vi "DecodeISAStatus.vi"(8 "error in (no error)":errorcluster, 11 "Message":string) -> (0 "error out":errorcluster, 1 "output cluster":T1, 2 "Pressure":dbl, 3 "IMP":i32, 5 "PWM":i32)   [LabVIEW 2017]
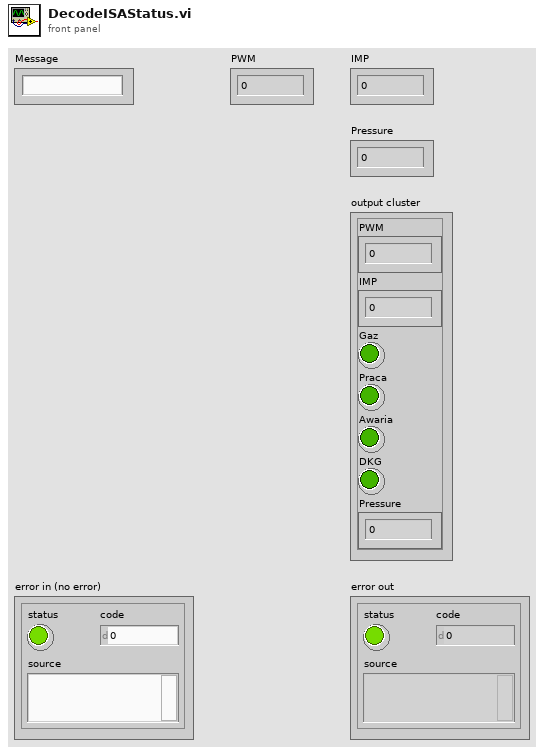
[diagram p1: front panel]
types:
  T1 = cluster{"PWM":i32, "IMP":i32, "Gaz":bool, "Praca":bool, "Awaria":bool, "DKG":bool, "Pressure":dbl}
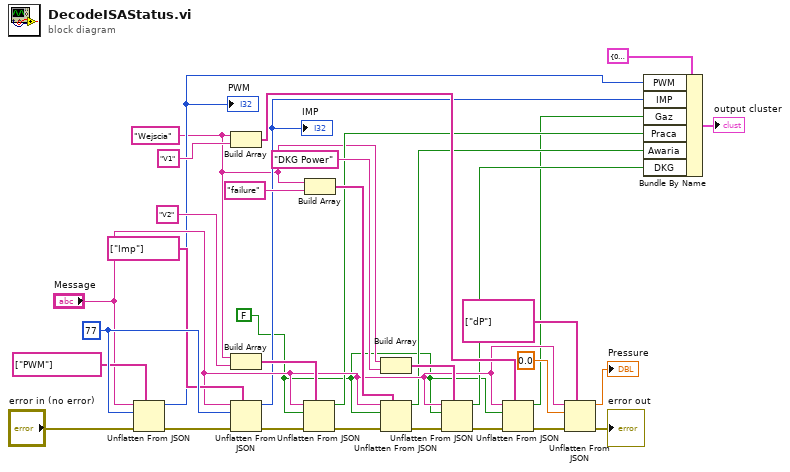
[diagram p0: block diagram]
diagram:
  w1 = FALSE
  w2 = "Wejscia"
  w30 = 77
  n1 = Unflatten From JSON(path=string[] ["PWM"], JSON string="Message", type and defaults=w30, error in (no error)="error in (no error)") -> (value=w11:i32, error out=w27:errorcluster)  [unwired: 3 in]
  "PWM" <- w11
  n2 = Build Array(w2, "V1" ("element")) -> (w14:string[])
  n3 = Build Array(w2, "V2" ("element")) -> (w17:string[])
  n4 = Unflatten From JSON(path=string[] ["Imp"], JSON string="Message", type and defaults=w30, error in (no error)=w27) -> (value=w10:i32, error out=w29:errorcluster)  [unwired: 3 in]
  "IMP" <- w10
  n5 = Unflatten From JSON(path=w17, JSON string="Message", type and defaults=w1, error in (no error)=w29) -> (value=w8:bool, error out=w25:errorcluster)  [unwired: 3 in]
  n6 = Build Array(w2, "failure" ("element")) -> (w16:string[])
  n7 = Build Array(w2, "DKG Power" ("element")) -> (w15:string[])
  n8 = Unflatten From JSON(path=w16, JSON string="Message", type and defaults=w1, error in (no error)=w25) -> (value=w7:bool, error out=w24:errorcluster)  [unwired: 3 in]
  n9 = Unflatten From JSON(path=w15, JSON string="Message", type and defaults=w1, error in (no error)=w24) -> (value=w6:bool, error out=w23:errorcluster)  [unwired: 3 in]
  n10 = Unflatten From JSON(path=w14, JSON string="Message", type and defaults=w1, error in (no error)=w23) -> (value=w5:bool, error out=w22:errorcluster)  [unwired: 3 in]
  n11 = Unflatten From JSON(path=string[] ["dP"], JSON string="Message", type and defaults=0.0, error in (no error)=w22) -> (value=→"Pressure":dbl, error out=→"error out":errorcluster)  [unwired: 3 in]
  n12 = Bundle By Name(cluster=T1 {"PWM"=0, "IMP"=0, "Gaz"=FALSE, "Praca"=FALSE, "Awaria"=FALSE, "DKG"=FALSE, "Pressure"=0.0} ("input cluster"), "PWM"=w11, "IMP"=w10, "Gaz"=w5, "Praca"=w8, "Awaria"=w7, "DKG"=w6) -> (→"output cluster":T1)
